vi "ArmExtend.vi"() -> ()   [LabVIEW 2018]
panel:
  in  "ArmExtend":bool
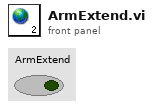
[diagram p1: front panel]
diagram:
